vi "hw7p6_hickey.vi"() -> ()   [LabVIEW 2014]
uses:
  <vilib>/MakerHub/LINX/Private/Type Defs/User Platform.ctl
  <vilib>/MakerHub/LINX/Private/Type Defs/Interface.ctl
  <vilib>/MakerHub/LINX/Public/Peripherals/Digital/Digital Write 1 Chan.vi
  <vilib>/MakerHub/LINX/LMH-LINX.lvlib
panel:
  in  "y":i32=5
  out "Error Out 2":errorcluster
  in  "milliseconds to wait":u32
  in  "DO Channel":u8
  out "Error Out":errorcluster
  in  "Serial Port":refnum<visa-resource-name>="N/A"
  in  "Interface":T1
  in  "Platform":T2
  in  "stop":bool
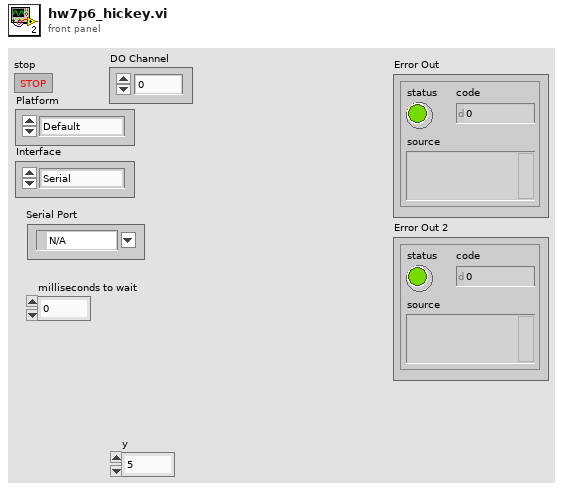
[diagram p1: front panel]
types:
  T1 = typedef "LMH-LINX.lvlib/Interface.ctl" = enum16{"Serial", "TCP"}
  T2 = typedef "LMH-LINX.lvlib/User Platform.ctl" = enum16{"Default", "LINX", "myRIO"}
  T3 = typedef "LMH-LINX.lvlib/LINX Ref.ctl" = cluster{"Platform":T4, "Interface":T1, "LINX Device Config":T5}
  T4 = typedef "LMH-LINX.lvlib/Platform.ctl" = enum16{"LINX", "myRIO"}
  T5 = typedef "LMH-LINX.lvlib/Device.lvlib/LINX Device Config.ctl" = cluster{"Interface":T1, "COM Port":refnum<visa-resource-name>, "TCP Configuration":T6, "Device Family":u8, "Device ID":u8, "Device Name":string, "TCP Ref":refnum<k5>, "Channels":T7}
  T6 = typedef "LMH-LINX.lvlib/Device.lvlib/TCP Config.ctl" = cluster{"IP Address":string, "Port":u16}
  T7 = typedef "LMH-LINX.lvlib/Channels.ctl" = cluster{"DI":u8[], "DO":u8[], "AI":u8[], "AO":u8[], "PWM":u8[], "QE":u8[], "UART":u8[], "I2C 2":u8[], "SPI":u8[], "CAN":u8[], "Servo":u8[], "AI Ref (V)":dbl, "AO Ref (V)":dbl, "AO Resolution (Bits)":u8}
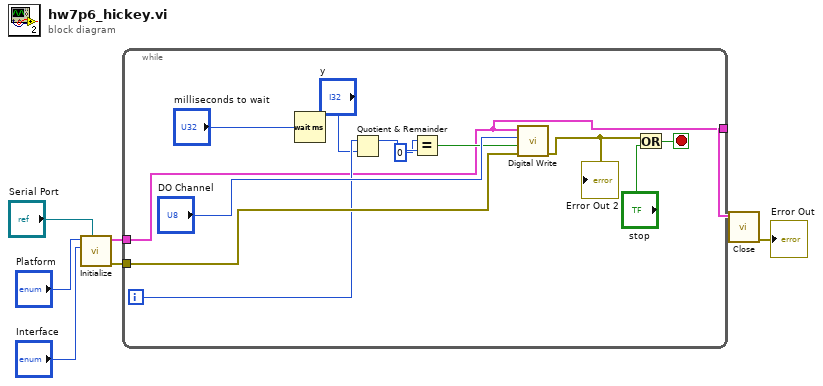
[diagram p0: block diagram]
diagram:
  n1 = call <vilib>:"Initialize.vi"("Serial Port"="Serial Port", "Interface"="Interface", "Platform"="Platform") -> ("Error Out"=w4:errorcluster, "LINX Ref"=w2:T3)  [unwired: 6 in, 1 out]
  n2 = while {
    tunnel: w4 -> [w14]
    tunnel: w2 -> [w9]
    tunnel: [w9] -> w1
    i -> [w10]
    stop <- w18 stop-if-true
    n3 = Wait (ms)(milliseconds to wait="milliseconds to wait") -> ()  [unwired: 1 out]
    n4 = Quotient & Remainder(x=w10, y="y") -> (x-y*floor(x/y)=w17:i32)  [unwired: 1 out]
    n5 = Equal?(x=u32 0 ("y"), y=w17) -> (x = y?=w13:bool)
    n6 = call-poly <vilib>:"Digital Write.vi"("Error In"=w14, "Output Value"=w13, "DO Channel"="DO Channel", "LINX Resource"=w9) -> ("Error Out"=w12:errorcluster)  [unwired: 6 in, 1 out]
    "Error Out 2" <- w12
    n7 = Or(x=w12, y="stop") -> (x .or. y?=w18:bool)
  }
  n8 = call <vilib>:"Close.vi"("LINX Resource"=w1) -> ("Error Out"=→"Error Out":errorcluster)  [unwired: 9 in, 1 out]
